vi "Init.vi"(7 "Level":T1, 8 "error in":errorcluster, 9 "Error to Log":errorcluster, 10 "Message":string, 11 "LogRecord in":refnum<class "LogRecord.lvclass">) -> (0 "error out":errorcluster, 3 "LogRecord out":refnum<class "LogRecord.lvclass">)   [LabVIEW 2016, in "hse-logger.lvlib" / "LogRecord.lvclass"]
doc: "Initilize a LogRecord object."
uses:
  LogRecord.lvclass
  LogLevel.ctl
  LogRecord.lvclass/LogRecord.ctl
  hse-logger.lvlib
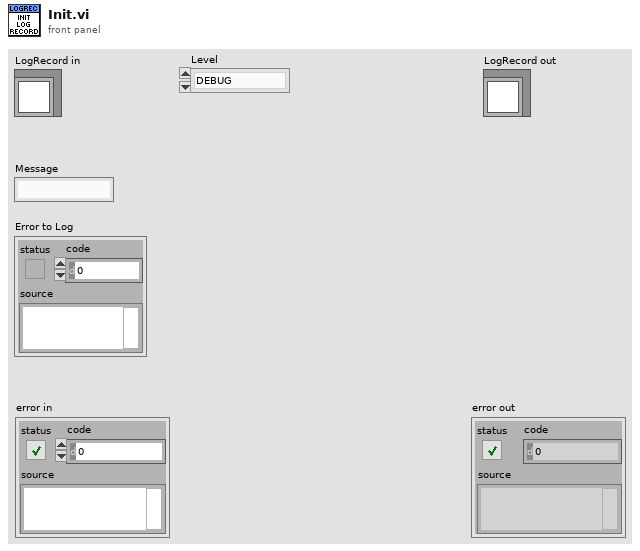
[diagram p1: front panel]
types:
  T1 = typedef "hse-logger.lvlib/LogLevel.ctl" = enum16{"DEBUG", "INFO", "WARNING", "ERROR", "CRITICAL"}
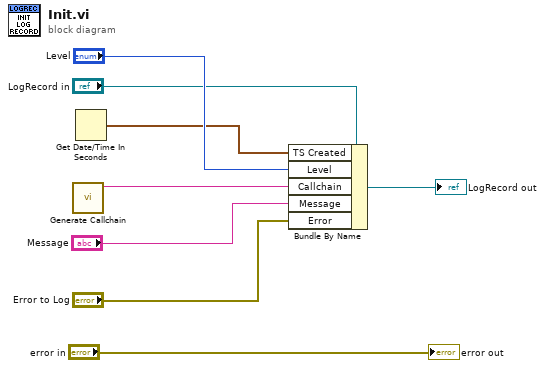
[diagram p0: block diagram]
diagram:
  n1 = call "Generate Callchain.vi"() -> ("Callchain"=w4:string)  [unwired: 11 in]
  n2 = Get Date/Time In Seconds() -> (seconds since 1Jan1904=w5:timestamp)
  n3 = Bundle By Name(cluster="LogRecord in", "TS Created"=w5, "Level"="Level", "Callchain"=w4, "Message"="Message", "Error"="Error to Log") -> (→"LogRecord out":refnum<class "LogRecord.lvclass">)
  "error out" <- "error in"
